vi "_SparkGetError.vi"(0 "AS Status":string, 1 "Oven Status":string, 2 "Pump 1 Status":string, 3 "Pump 2 Status":string, 4 "LC Status":string) -> (5 "LC Error":string)   [LabVIEW 2012]
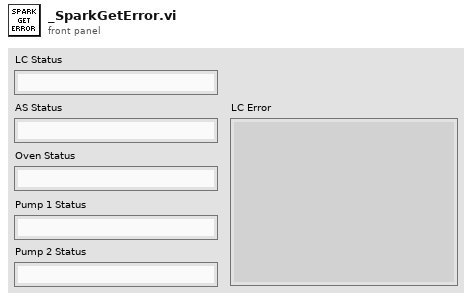
[diagram p1: front panel]
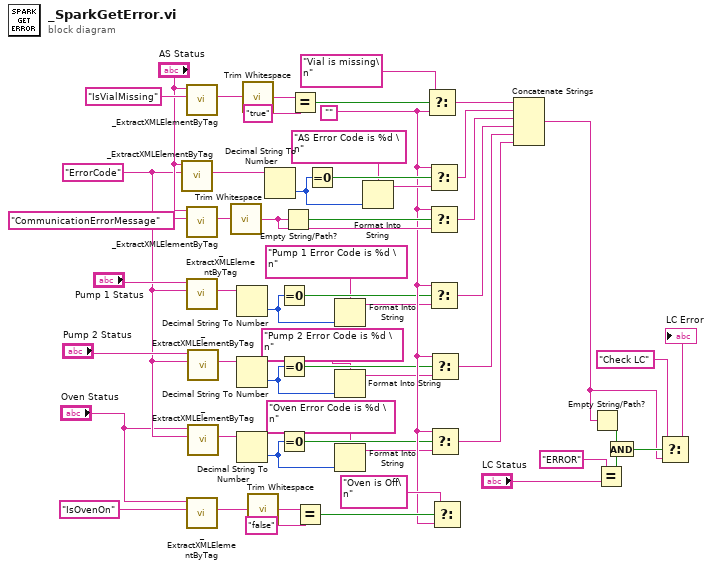
[diagram p0: block diagram]
diagram:
  w25 = ""
  w40 = "ErrorCode" ("TagName")
  n1 = call "_ExtractXMLElementByTag.vi"("TagName"=w40, "XML String"="AS Status") -> ("Element"=w29:string)  [unwired: 2 in, 3 out]
  n2 = call "_ExtractXMLElementByTag.vi"("TagName"="IsVialMissing", "XML String"="AS Status") -> ("Element"=w55:string)  [unwired: 2 in, 3 out]
  n3 = call "_ExtractXMLElementByTag.vi"("TagName"="CommunicationErrorMessage", "XML String"="AS Status") -> ("Element"=w50:string)  [unwired: 2 in, 3 out]
  n4 = call "_ExtractXMLElementByTag.vi"("TagName"=w40, "XML String"="Pump 1 Status") -> ("Element"=w23:string)  [unwired: 2 in, 3 out]
  n5 = call "_ExtractXMLElementByTag.vi"("TagName"="IsOvenOn", "XML String"="Oven Status") -> ("Element"=w37:string)  [unwired: 2 in, 3 out]
  n6 = call "_ExtractXMLElementByTag.vi"("TagName"=w40, "XML String"="Pump 2 Status") -> ("Element"=w18:string)  [unwired: 2 in, 3 out]
  n7 = call "_ExtractXMLElementByTag.vi"("TagName"=w40, "XML String"="Oven Status") -> ("Element"=w14:string)  [unwired: 2 in, 3 out]
  n8 = call <vilib>:"Trim Whitespace.vi"("string"=w50) -> ("trimmed string"=w31:string)  [unwired: 1 in]
  n9 = Decimal String To Number(string=w23) -> (number=w24:i32)  [unwired: 2 in, 1 out]
  n10 = Decimal String To Number(string=w18) -> (number=w19:i32)  [unwired: 2 in, 1 out]
  n11 = Decimal String To Number(string=w14) -> (number=w15:i32)  [unwired: 2 in, 1 out]
  n12 = call <vilib>:"Trim Whitespace.vi"("string"=w55) -> ("trimmed string"=w54:string)  [unwired: 1 in]
  n13 = call <vilib>:"Trim Whitespace.vi"("string"=w37) -> ("trimmed string"=w44:string)  [unwired: 1 in]
  n14 = Decimal String To Number(string=w29) -> (number=w30:i32)  [unwired: 2 in, 1 out]
  n15 = Equal To 0?(x=w24) -> (x = 0?=w22:bool)
  n16 = Equal To 0?(x=w19) -> (x = 0?=w17:bool)
  n17 = Equal To 0?(x=w15) -> (x = 0?=w13:bool)
  n18 = Empty String/Path?(string/path=w31) -> (empty?=w47:bool)
  n19 = Equal?(x=w54, y="true") -> (x = y?=w52:bool)
  n20 = Equal?(x=w44, y="false") -> (x = y?=w42:bool)
  n21 = Equal To 0?(x=w30) -> (x = 0?=w28:bool)
  n22 = Format Into String(format string="Pump 1 Error Code is %d \n", w24) -> (resulting string=w20:string)  [unwired: 2 in, 1 out]
  n23 = Format Into String(format string="Pump 2 Error Code is %d \n", w19) -> (resulting string=w10:string)  [unwired: 2 in, 1 out]
  n24 = Format Into String(format string="Oven Error Code is %d \n", w15) -> (resulting string=w11:string)  [unwired: 2 in, 1 out]
  n25 = Format Into String(format string="AS Error Code is %d \n", w30) -> (resulting string=w26:string)  [unwired: 2 in, 1 out]
  n26 = Select(t="Vial is missing\n", s=w52, f=w25) -> (s? t:f=w36:string)
  n27 = Select(t=w25, s=w28, f=w26) -> (s? t:f=w35:string)
  n28 = Select(t=w25, s=w47, f=w31) -> (s? t:f=w34:string)
  n29 = Select(t=w25, s=w22, f=w20) -> (s? t:f=w33:string)
  n30 = Select(t=w25, s=w17, f=w10) -> (s? t:f=w9:string)
  n31 = Select(t=w25, s=w13, f=w11) -> (s? t:f=w32:string)
  n32 = Select(t="Oven is Off\n", s=w42, f=w25) -> ()  [unwired: 1 out]
  n33 = Concatenate Strings(w36, w35, w34, w33, w9, w32) -> (w2:string)
  n34 = Empty String/Path?(string/path=w2) -> (empty?=w6:bool)
  n35 = Equal?(x="ERROR", y="LC Status") -> (x = y?=w7:bool)
  n36 = And(x=w6, y=w7) -> (x .and. y?=w5:bool)
  n37 = Select(t="Check LC" ("f"), s=w5, f=w2) -> (s? t:f=→"LC Error":string)
